vi "Ejercicio 1. 2.vi"() -> ()   [LabVIEW 2021]
panel:
  out "Numeric":dbl
  out "`[0.75, 1]":bool
  out "[0.5, 0.75]":bool
  out "[0.25 , 0.5]":bool
  out "[0 , 0.25]":bool
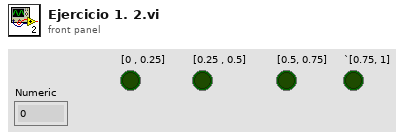
[diagram p1: front panel]
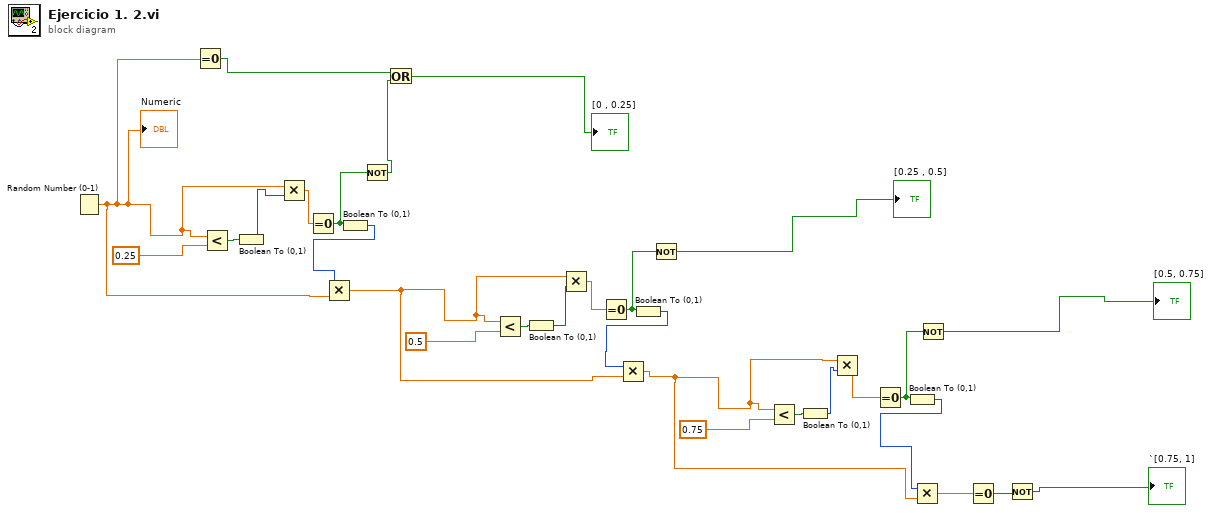
[diagram p0: block diagram]
diagram:
  n1 = Random Number (0-1)() -> (number: 0 to 1=w4:dbl)
  "Numeric" <- w4
  n2 = Equal To 0?(x=w4) -> (x = 0?=w3:bool)
  n3 = Less?(x=w4, y=0.25) -> (x < y?=w29:bool)
  n4 = Boolean To (0,1)(Boolean=w29) -> (0, 1=w20:i16)
  n5 = Multiply(x=w4, y=w20) -> (x*y=w19:dbl)
  n6 = Equal To 0?(x=w19) -> (x = 0?=w24:bool)
  n7 = Boolean To (0,1)(Boolean=w24) -> (0, 1=w14:i16)
  n8 = Multiply(x=w14, y=w4) -> (x*y=w13:dbl)
  n9 = Not(x=w24) -> (.not. x?=w2:bool)
  n10 = Or(x=w3, y=w2) -> (x .or. y?=→"[0 , 0.25]":bool)
  n11 = Less?(x=w13, y=0.5) -> (x < y?=w27:bool)
  n12 = Boolean To (0,1)(Boolean=w27) -> (0, 1=w18:i16)
  n13 = Multiply(x=w13, y=w18) -> (x*y=w17:dbl)
  n14 = Equal To 0?(x=w17) -> (x = 0?=w23:bool)
  n15 = Boolean To (0,1)(Boolean=w23) -> (0, 1=w12:i16)
  n16 = Multiply(x=w12, y=w13) -> (x*y=w10:dbl)
  n17 = Not(x=w23) -> (.not. x?=→"[0.25 , 0.5]":bool)
  n18 = Less?(x=w10, y=0.75) -> (x < y?=w25:bool)
  n19 = Boolean To (0,1)(Boolean=w25) -> (0, 1=w16:i16)
  n20 = Multiply(x=w10, y=w16) -> (x*y=w15:dbl)
  n21 = Equal To 0?(x=w15) -> (x = 0?=w22:bool)
  n22 = Boolean To (0,1)(Boolean=w22) -> (0, 1=w11:i16)
  n23 = Multiply(x=w11, y=w10) -> (x*y=w9:dbl)
  n24 = Not(x=w22) -> (.not. x?=→"[0.5, 0.75]":bool)
  n25 = Equal To 0?(x=w9) -> (x = 0?=w8:bool)
  n26 = Not(x=w8) -> (.not. x?=→"`[0.75, 1]":bool)
